vi "Fpga.vi"() -> ()   [LabVIEW 2019]
uses:
  <vilib>/rvi/Emulation/niFpgaGetClockAttributes.vi
  <vilib>/rvi/Emulation/niFpgaSctlEmulationGetInTimedLoop.vi
  <vilib>/rvi/Emulation/niFpgaEmulationReportErrorSimple.vi
  <vilib>/rvi/eio/common/nirviEmuTemplateMethod_errors.vi
  <vilib>/rvi/interface/RandomDataEmulation/niFpgaRandomDataHandleErrors.vi
  <vilib>/rvi/Emulation/niFpgaCriticalErrorInLSC.vi
  <vilib>/eio/EIONode/EIONode.xnode
  <vilib>/rvi/DataTransferAndStorage/Container/XNode/niFpgaContainer.xnode
  <vilib>/rvi/interface/RandomDataEmulation/nirviRandomDataFpgaReadWriteTemplate.vi
panel:
  in  "Voltage In":fxp<+/-,20,5>
  out "Voltage Out":fxp<+/-,20,5>
  out "Timed Out?":bool
  in  "Position Reset":bool
  in  "stop 2":bool
  out "Position (Counts)":i32
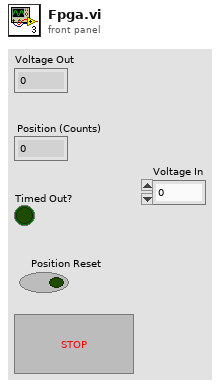
[diagram p1: front panel]
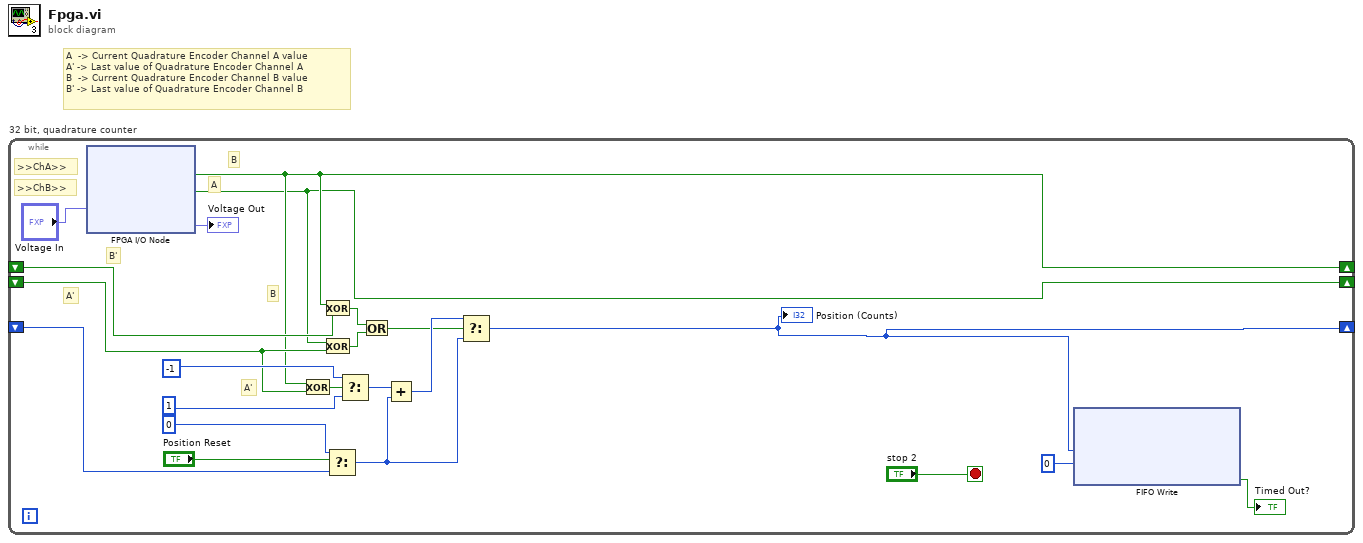
[diagram p0: block diagram]
diagram:
  # "A  -> Current Quadrature Encoder Channel A value\nA' -> Last value of Quadrature Encoder Channel A\nB  -> Current Quadrature Encoder Channel B value\nB' -> Last value of Quadrature Encoder Channel B"
  n1 = while "32 bit, quadrature counter" {
    shift-right: [w7] -> _
    shift-left: _ -> [w8]
    shift-right: [w2] -> _
    shift-left: _ -> [w9]
    shift-right: [w6] -> _
    shift-left: _ -> [w12]
    stop <- "stop 2" stop-if-true
    # ">>ChB>>"
    # ">>ChA>>"
    # "A'"
    # "B"
    # "A'"
    # "A"
    # "B'"
    # "B"
    n2 = xnode "FPGA I/O Node"("Mod3/AO0"="Voltage In") -> ("Mod1/DI0"=w7:bool, "Mod1/DI1"=w6:bool, "Mod4/AI0"=→"Voltage Out":fxp<+/-,20,5>)  [unwired: 4 in, 4 out]
    n3 = Exclusive Or(1:w12, 2:w7) -> (0:w13:bool)
    n4 = Exclusive Or(1:w8, 2:w7) -> (0:w14:bool)
    n5 = Exclusive Or(1:w12, 2:w6) -> (0:w15:bool)
    n6 = Select(t=0 ("32 bit"), s="Position Reset", f=w9) -> (s? t:f=w20:i32)
    n7 = Select(t=-1 ("32 bit"), s=w13, f=1 ("32 bit")) -> (s? t:f=w18:i32)
    n8 = Or(x=w14, y=w15) -> (x .or. y?=w10:bool)
    n9 = Add(x=w18, y=w20) -> (x+y=w22:i32)
    n10 = Select(t=w22, s=w10, f=w20) -> (s? t:f=w2:i32)
    "Position (Counts)" <- w2
    n11 = xnode ("FIFO Write")("Element"=w2, "Timeout"=0) -> ("Timed Out?"=→"Timed Out?":bool)  [unwired: 1 in, 1 out]
  }
